vi "F Dwf Digital In Input Order Set.vi"(8 "error in (no error)":errorcluster, 10 "fDioFirst":bool, 11 "hdwf":i32) -> (0 "error out":errorcluster, 3 "function return":i32)   [LabVIEW 2019, in "Olasdwf.lvlib"]
doc: "DWFAPI int FDwfDigitalInInputOrderSet(HDWF hdwf, bool fDioFirst);"
uses:
  Olasdwf.lvlib
  Windows/System32/dwf.dll
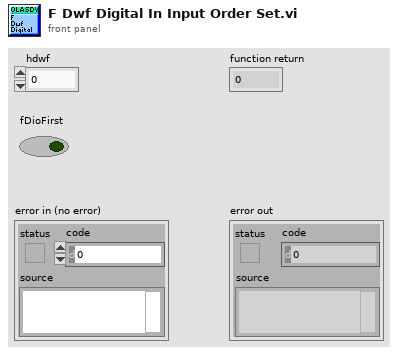
[diagram p1: front panel]
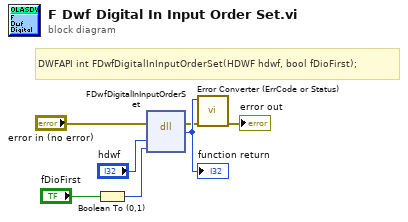
[diagram p0: block diagram]
diagram:
  # "DWFAPI int FDwfDigitalInInputOrderSet(HDWF hdwf, bool fDioFirst);"
  n1 = Boolean To (0,1)(Boolean="fDioFirst") -> (0, 1=w4:i16)
  n2 = dll-call lib="C:/Windows/System32/dwf.*" fn="FDwfDigitalInInputOrderSet"(error in="error in (no error)", "hdwf"="hdwf", "fDioFirst"=w4) -> (error out=w2:errorcluster, w7:i32)  [unwired: 4 in, 1 out]
  "function return" <- w7
  n3 = call "Error Converter (ErrCode or Status).vi"("error in (no error)"=w2, "error code"=w7) -> ("error out"=→"error out":errorcluster)  [unwired: 9 in]
